vi "Estimate_State-Space_Model_from_FRFs_Iteractive_Parameter_Adjustment_v0.vi"() -> ()   [LabVIEW 2022 SP3]
doc: "This example demonstrates how to use frequency-domain data to estimate a state-space model. \n\n<B>Instructions:</B>\n1) Run this VI.\n2) Observe how the simulated frequency response matches the measured frequency response.\n3) Change the orders of the models, and observe how these changes affect the estimation error."
uses:
  <vilib>/addons/System Identification/Model Typedefs.llb/SI Pole-Zero Plot.ctl
  <vilib>/addons/System Identification/Frequency Domain Estimation.llb/SI Estimate Discrete State-Space Model from FRF (SISO Arbitrary).vi
  <vilib>/addons/System Identification/NI_SysID.lvlib
  <vilib>/Analysis/NI_AALPro.lvlib
panel:
  in  "Max. Noise\nSubspace":i32=80
  in  "Max. Order":i32=8
  out "Current Order":i32
  out "Currrent Noise":i32
  out "Current Error":dbl format="%0.2f"
  in  "milliseconds to wait":u32=125
  out "Cluster":cluster{"Order":i32, "Noise Subspace":i32}
  out "Lowest Error":i32
  in  "confidence level (%)":dbl=99.0 format="%_2f"
  out "pole-zero plot":T1
  in  "name or relative path":path=path "C:/Users/LAV-UFSC/OneDrive - UFSC/Documents/LAV - TCC/Dados-Experimentos/25-04/frf_2.txt"
  in  "FRF format":T2={"dB on? (F)"=FALSE, "unwrap phase? (F)"=FALSE, "convert to degree? (F)"=TRUE}
  out "Phase Response":cluster{"frequency":dbl[], "amplitude":dbl[]}[](graph)
  out "Magnitude Response":cluster{"frequency":dbl[], "amplitude":dbl[]}[](graph)
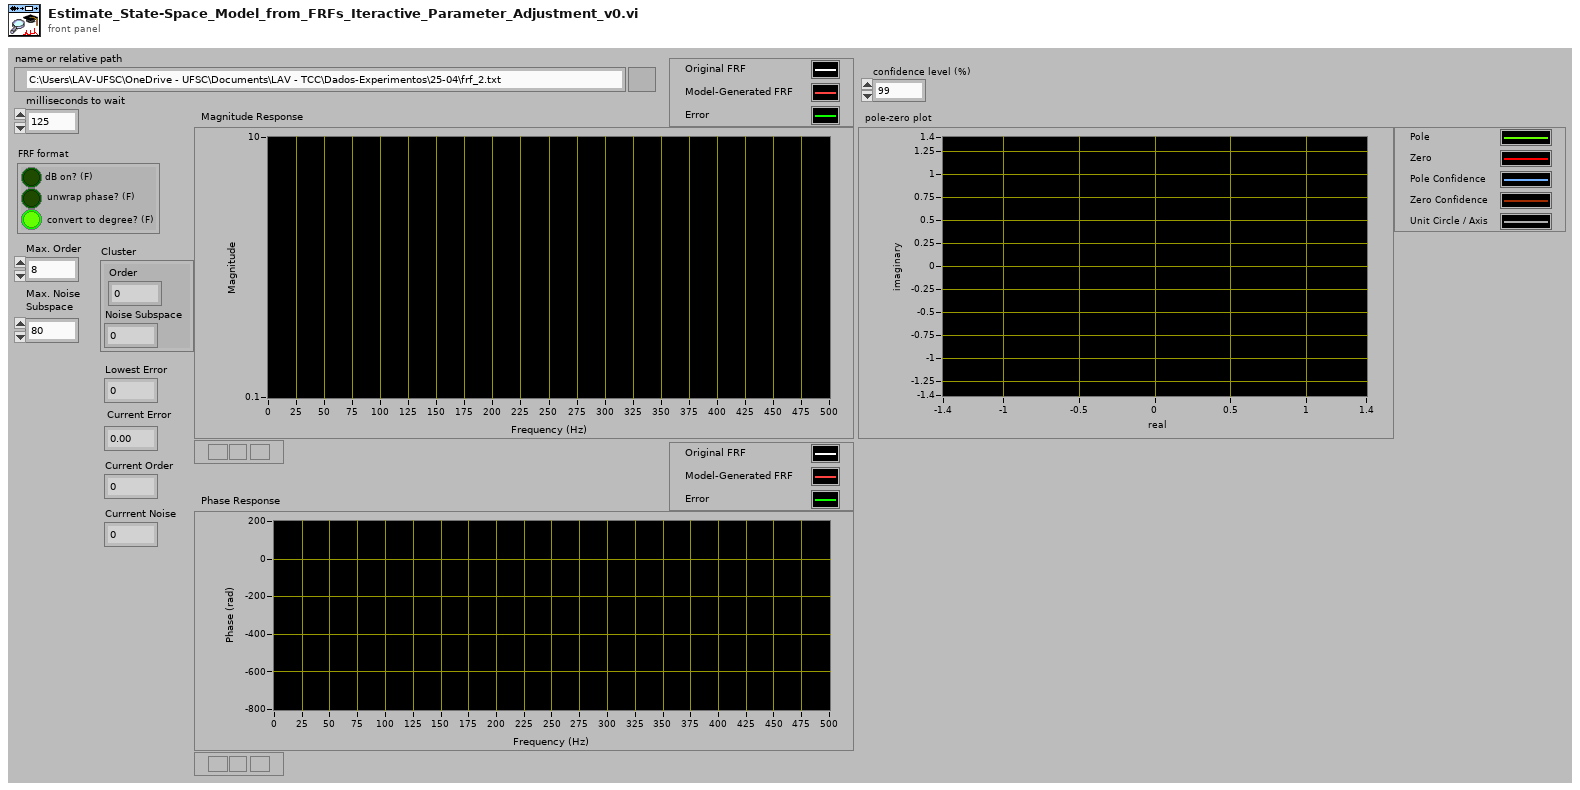
[diagram p1: front panel]
types:
  T1 = typedef "NI_SysID.lvlib/SI Pole-Zero Plot.ctl" = cluster{"frequency":dbl[], "amplitude":dbl[]}[]
  T2 = cluster{"dB on? (F)":bool, "unwrap phase? (F)":bool, "convert to degree? (F)":bool}
  T3 = cluster{"start frequency":dbl, "end frequency":dbl, "num of freq bins":i32, "interval type":u16}
  T4 = typedef "NI_SysID.lvlib/si_generic model.ctl" = cluster{"attributes":cluster{"version":string, "model type":T5, "input names":string[], "output names":string[], "notes":string}, "coefficients":cluster{"A ":dbl[][][], "B":dbl[][][], "F":dbl[][][], "C":dbl[][][], "D":dbl[][][]}, "std deviations":cluster{"A ":dbl[][][], "B":dbl[][][], "F":dbl[][][], "C":dbl[][][], "D":dbl[][][]}, "coefficients covariance":dbl[][][], "noise variance":dbl[][], "fs":dbl, "system info":cluster{"number of inputs":i32, "number of outputs":i32, "A order":i32[][], "B order":i32[][], "F order":i32[][], "C order":i32[][], "D order":i32[][], "Delays":i32[][]}, "kalman gain":dbl[][], "initial state":dbl[], "trans func":cluster{"betas":dbl[], "alphas":dbl[]}[][], "zeros-poles":cluster{"zeros":cdb[], "poles":cdb[], "gain":dbl}[][], "std of trans func":cluster{"betas":dbl[], "alphas":dbl[]}[][], "std of zeros-poles":cluster{"zeros":cdb[], "poles":cdb[], "gain":dbl}[][], "trans func (noise)":cluster{"betas":dbl[], "alphas":dbl[]}[][], "std of trans func (noise)":cluster{"betas":dbl[], "alphas":dbl[]}[][], "zeros-poles (noise)":cluster{"zeros":cdb[], "poles":cdb[], "gain":dbl}[][], "std of zeros-poles (noise)":cluster{"zeros":cdb[], "poles":cdb[], "gain":dbl}[][], "Symbolic State Space Model":cluster{"Symbolic A":string[][], "Symbolic B":string[][], "Symbolic C":string[][], "Symbolic D":string[][], "Symbolic K":string[][], "Symbolic Initial State":string[]}, "delay":dbl[][], "variables":T6, "grey trans func spec":cluster{"orders of TF model":cluster{" num order":i32, "den order":i32}, "# of zeros/poles at origin":cluster{"zeros/poles":u16, "number ":i32}, "delay initial?":bool, "gain initial?":bool}}
  T5 = typedef "NI_SysID.lvlib/SI Model Type.ctl" = u16
  T6 = typedef "NI_SysID.lvlib/si_variables.ctl" = cluster{"name":string, "initial guess":dbl, "upper limit":dbl, "lower limit":dbl, "value":dbl}[]
  T7 = typedef "NI_SysID.lvlib/si_Bode Phase Plot.ctl" = cluster{"frequency":dbl[], "amplitude":dbl[]}[]
  T8 = typedef "NI_SysID.lvlib/si_Bode Magnitude Plot.ctl" = cluster{"frequency":dbl[], "amplitude":dbl[]}[]
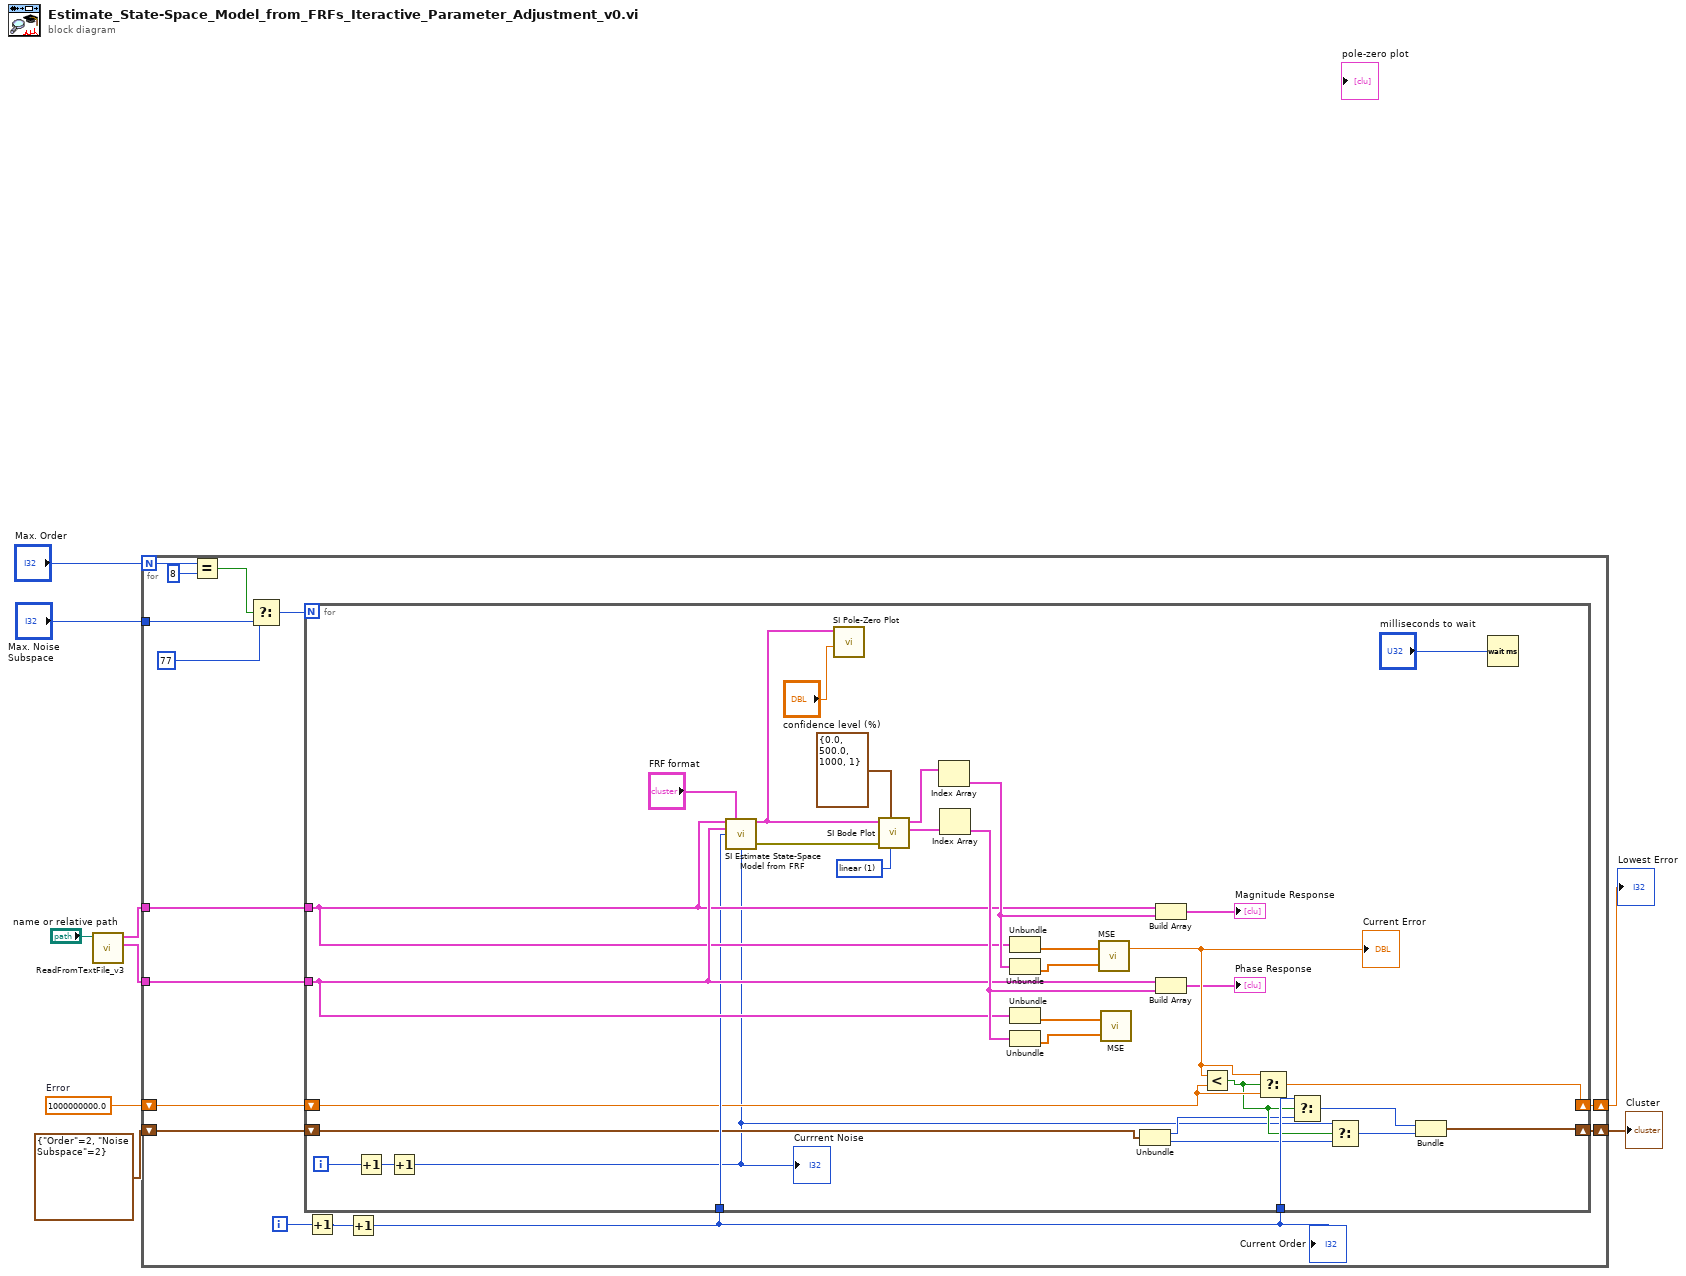
[diagram p0: block diagram]
diagram:
  w5 = 1000000000.0  # Error
  n1 = call "ReadFromTextFile_v3.vi"("name or relative path"="name or relative path") -> ("Phase"=w7:cluster{dbl[], dbl[]}, "Magnitude"=w6:cluster{dbl[], dbl[]})  [unwired: 6 in, 2 out]
  n2 = for {
    N: "Max. Order" -> [w15]
    tunnel: w7 -> [w24]
    tunnel: w6 -> [w23]
    shift-right: [w21] -> w4
    shift-left: w5 -> [w22]
    shift-right: [w20] -> w2
    shift-left: cluster{"Order":i32, "Noise Subspace":i32} {"Order"=2, "Noise Subspace"=2} -> [w19]
    tunnel: "Max. Noise\nSubspace" -> [w10]
    i -> [w18]
    n3 = Equal?(x=w15, y=8) -> (x = y?=w12:bool)
    n4 = Select(t=77, s=w12, f=w10) -> (s? t:f=w13:i32)
    n5 = Increment(x=w18) -> (x+1=w17:i32)
    n6 = Increment(x=w17) -> (x+1=w16:i32)
    "Current Order" <- w16
    n7 = for {
      N: w13 -> [_]
      tunnel: w24 -> [w48]
      tunnel: w23 -> [w47]
      tunnel: w16 -> [w46]
      shift-right: [w39] -> w21
      shift-left: w22 -> [w40]
      shift-right: [w34] -> w20
      shift-left: w19 -> [w31]
      tunnel: w16 -> [w38]
      i -> [w30]
      w50 = u16 1 items=["dB", "linear"] ("magnitude unit")
      n8 = Increment(x=w30) -> (x+1=w29:i32)
      n9 = Increment(x=w29) -> (x+1=w25:i32)
      "Currrent Noise" <- w25
      n10 = call-poly <vilib>:"SI Estimate State-Space Model from FRF.vi"("FRF magnitude"=w47, "FRF format"="FRF format", "FRF phase"=w48, "number of states"=w46, "noise subspace (%)"=w25) -> ("system model out"=w53:T4, "error out"=w52:errorcluster)  [unwired: 3 in, 6 out]
      n11 = call <vilib>:"SI Pole-Zero Plot.vi"("confidence level (%)"="confidence level (%)", "system model"=w53) -> ()  [unwired: 8 in, 2 out]
      n12 = call <vilib>:"SI Bode Plot.vi"("magnitude unit"=w50, "freq info"=T3 {"start frequency"=0.0, "end frequency"=500.0, "num of freq bins"=1000, "interval type"=1}, "error in (no error)"=w52, "system model"=w53) -> ("Bode phase plot"=w56:T7, "Bode magnitude plot"=w55:T8)  [unwired: 3 in, 3 out]
      n13 = Index Array(array=w55) -> (element=w58:cluster{"frequency":dbl[], "amplitude":dbl[]})  [unwired: 1 in]
      n14 = Index Array(array=w56) -> (element=w57:cluster{"frequency":dbl[], "amplitude":dbl[]})  [unwired: 1 in]
      n15 = Unbundle(w47) -> (w45:dbl[])  [unwired: 1 out]
      n16 = Unbundle(w58) -> ("amplitude"=w44:dbl[])  [unwired: 1 out]
      n17 = Unbundle(w48) -> (w43:dbl[])  [unwired: 1 out]
      n18 = Unbundle(w57) -> ("amplitude"=w42:dbl[])  [unwired: 1 out]
      n19 = call <vilib>:"MSE.vi"("X Values"=w44, "Y Values"=w45) -> ("mse"=w41:dbl)  [unwired: 1 out]
      "Current Error" <- w41
      n20 = call <vilib>:"MSE.vi"("X Values"=w42, "Y Values"=w43) -> ()  [unwired: 2 out]
      n21 = Unbundle(w31) -> ("Order"=w33:i32, "Noise Subspace"=w32:i32)
      n22 = Build Array(w47, w58) -> (→"Magnitude Response":cluster{"frequency":dbl[], "amplitude":dbl[]}[])
      n23 = Build Array(w48, w57) -> (→"Phase Response":cluster{"frequency":dbl[], "amplitude":dbl[]}[])
      n24 = Less?(x=w41, y=w40) -> (x < y?=w37:bool)
      n25 = Select(t=w41, s=w37, f=w40) -> (s? t:f=w39:dbl)
      n26 = Select(t=w38, s=w37, f=w33) -> (s? t:f=w36:i32)
      n27 = Select(t=w25, s=w37, f=w32) -> (s? t:f=w35:i32)
      n28 = Bundle("Order"=w36, "Noise Subspace"=w35) -> (w34:cluster{"Order":i32, "Noise Subspace":i32})  [unwired: 1 in]
      n29 = Wait (ms)(milliseconds to wait="milliseconds to wait") -> ()  [unwired: 1 out]
    }
  }
  "Lowest Error" <- w4
  "Cluster" <- w2
